vi "update sync names.vi"(8 "error in":errorcluster, 10 "engine in":refnum<class "Engine Parent Editor Node.lvclass">, 11 "shared memory editor node in":refnum<class "module editor node.lvclass">) -> (0 "error out":errorcluster, 2 "engine out":refnum<class "Engine Parent Editor Node.lvclass">, 3 "shared memory editor node out":refnum<class "module editor node.lvclass">)   [LabVIEW 2014, in "Shared Memory editor node.lvclass"]
uses:
  Shared Memory editor node.lvclass
  <vilib>/NI/DCAF/Tag Editor Core/Configuration Editor/Classes/Module editor node/module editor node.lvclass
  <vilib>/NI/DCAF/Tag Editor Core/Configuration Editor/Classes/Engine Parent/Engine Parent Editor Node.lvclass
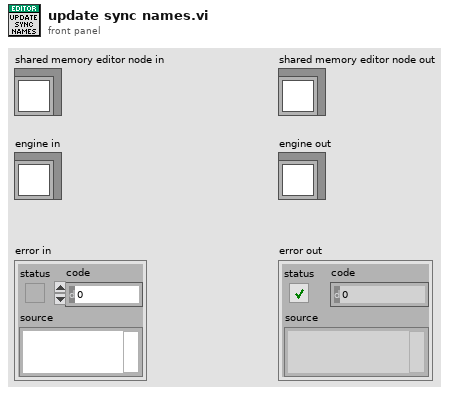
[diagram p1: front panel]
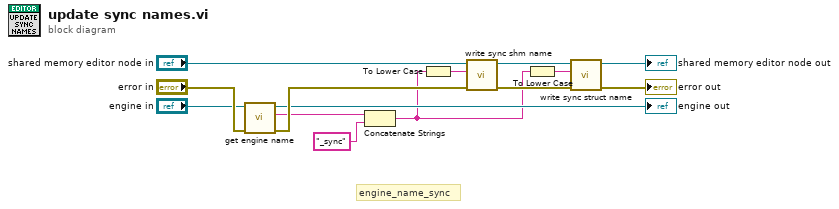
[diagram p0: block diagram]
diagram:
  # "engine_name_sync"
  n1 = call "get engine name.vi"("error in (no error)"="error in", "engine in"="engine in") -> ("error out"=w14:errorcluster, "engine name"=w1:string, "engine out"=→"engine out":refnum<class "Engine Parent Editor Node.lvclass">)  [unwired: 7 in]
  n2 = Concatenate Strings(w1, "_sync" ("string")) -> (w2:string)
  n3 = To Lower Case(string=w2) -> (all lower case string=w3:string)
  n4 = call "write sync shm name.vi"("error in"=w14, "shm name"=w3, "shared memory editor node"="shared memory editor node in") -> ("error out"=w7:errorcluster, "shared memory editor node out"=w9:refnum<class "module editor node.lvclass">)  [unwired: 7 in]
  n5 = To Lower Case(string=w2) -> (all lower case string=w4:string)
  n6 = call "write sync struct name.vi"("error in"=w7, "struct name"=w4, "shared memory editor node"=w9) -> ("error out"=→"error out":errorcluster, "shared memory editor node out"=→"shared memory editor node out":refnum<class "module editor node.lvclass">)  [unwired: 7 in]
